vi "Differential Drive Odometry - Delta Angle.vi"(6 "Reset":bool, 9 "Delta Theta":dbl, 10 "Right Distance":dbl, 11 "Left Distance":dbl) -> (3 "Pose":T1)   [LabVIEW 2019]
uses:
  <vilib>/Rock Robotics/WPI/ThirdParty/WPILib Extensions/Geometry/Typedef/Pose2d.ctl
  <vilib>/Rock Robotics/WPI/ThirdParty/WPILib Extensions/Geometry/Typedef/Translation2d.ctl
  <vilib>/Rock Robotics/WPI/ThirdParty/WPILib Extensions/Geometry/Typedef/Rotation2d.ctl
  <vilib>/Analysis/coordinate.llb/2D Cartesian Coordinate Rotation (Scalar).vi
  Odometry Set.vi
  <vilib>/Analysis/NI_AALPro.lvlib
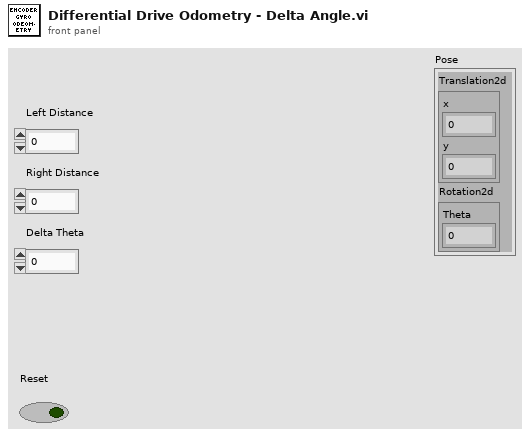
[diagram p1: front panel]
types:
  T1 = typedef "Pose2d.ctl" = cluster{"Translation2d":T2, "Rotation2d":T3}
  T2 = typedef "Translation2d.ctl" = cluster{"x":dbl, "y":dbl}
  T3 = typedef "Rotation2d.ctl" = cluster{"Theta":dbl}
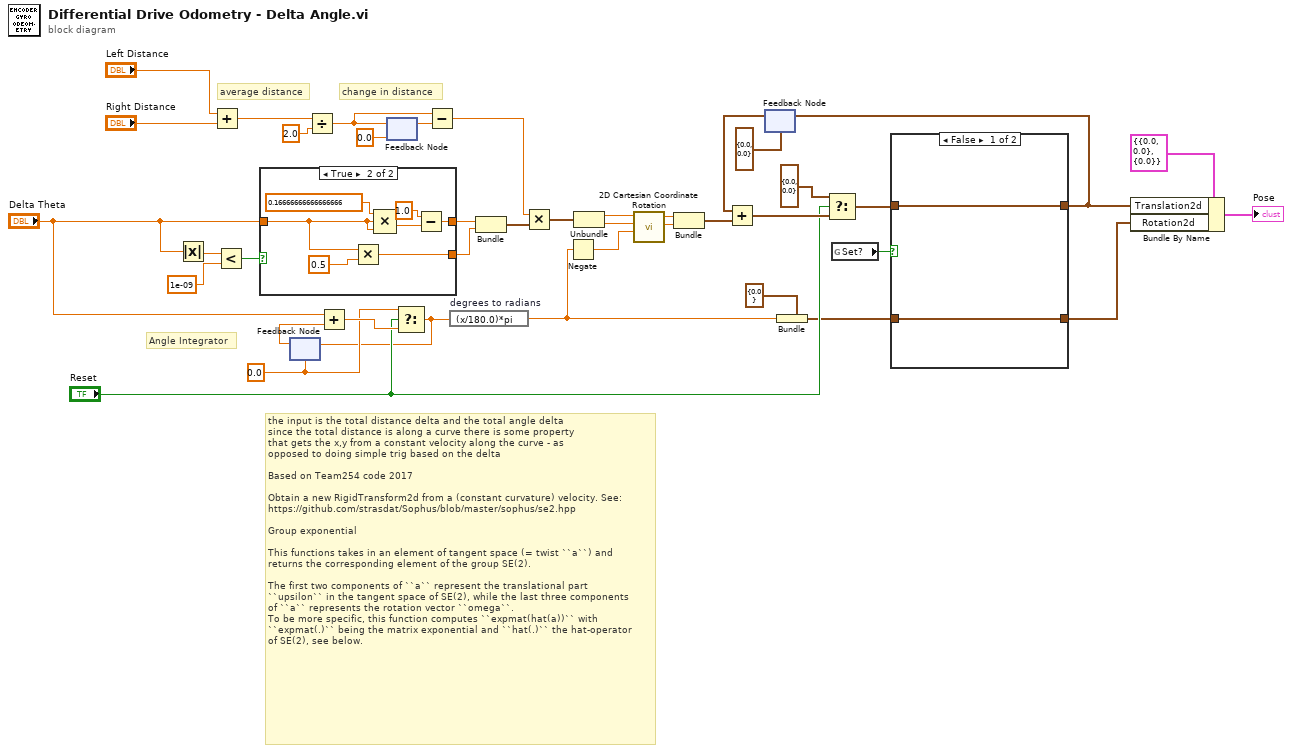
[diagram p0: block diagram]
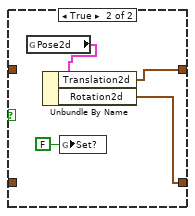
[diagram p2: hidden frame]
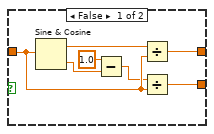
[diagram p3: hidden frame]
diagram:
  w9 = 0.0 ("Delta Theta")
  # "Angle Integrator"
  # "the input is the total distance delta and the total angle delta\nsince the total distance is along a curve there is some property \nthat gets the x,y from a constant velocity along the curve - as\nopposed to doing simple trig based on the delta\n\nBased on Team254 code 2017\n\nObtain a new RigidTransform2d from a (constant curvature) velocity. See:\nhttps://github.com/strasdat/Sophus/blob/master/sophus/se2.hpp\n\nGroup exponential\n\nThis functions takes in an element of tangent space (= twist ``a``) and\nreturns the corresponding element of the group SE(2).\n\nThe first two components of ``a`` represent the translational part\n``upsilon`` in the tangent space of SE(2), while the last three components\nof ``a`` represents the rotation vector ``omega``.\nTo be more specific, this function computes ``expmat(hat(a))`` with\n``expmat(.)`` being the matrix exponential and ``hat(.)`` the hat-operator\nof SE(2), see below."
  # "change in distance"
  # "average distance"
  n1 = Absolute Value(x="Delta Theta") -> (abs(x)=w31:dbl)
  n2 = Add(x="Left Distance", y="Right Distance") -> (x+y=w35:dbl)
  n3 = Less?(x=w31, y=1e-09) -> (x < y?=w29:bool)
  n4 = case shown="True" w29 {
    tunnel: "Delta Theta" -> [w46 w48]
    tunnel: [w42 w49] -> w28
    tunnel: [w41 w53] -> w27
    frame False {
      n5 = Sine & Cosine(0:w46) -> (1:w47:dbl, 2:w44:dbl)
      n6 = Subtract(x=1.0, y=w44) -> (x-y=w43:dbl)
      n7 = Divide(x=w47, y=w46) -> (x/y=w42:dbl)
      n8 = Divide(x=w43, y=w46) -> (x/y=w41:dbl)
    }
    frame True {
      n9 = Multiply(x=w48, y=0.5) -> (x*y=w53:dbl)
      n10 = Compound Arithmetic op=MULTIPLY(0.16666666666666666 ("y"), w48, w48) -> (w52:dbl)
      n11 = Subtract(x=1.0, y=w52) -> (x-y=w49:dbl)
    }
  }
  n12 = feedback #1(w9) -> (w12:dbl)
  n13 = Divide(x=w35, y=2.0) -> (x/y=w34:dbl)
  n14 = Add(x="Delta Theta", y=w12) -> (x+y=w10:dbl)
  n15 = feedback #2(0.0) -> (w40:dbl)
  n16 = feedback-in #2(w34) -> ()
  n17 = Select(t=w9, s="Reset", f=w10) -> (s? t:f=w7:dbl)
  n18 = feedback-in #1(w7) -> ()
  n19 = Subtract(x=w34, y=w40) -> (x-y=w25:dbl)
  n20 = expression code="(x/180.0)*pi" "degrees to radians"(w7) -> (w1:dbl)
  n21 = Bundle(w28, w27) -> (w26:cluster{dbl, dbl})  [unwired: 1 in]
  n22 = Multiply(x=w25, y=w26) -> (x*y=w24:cluster{dbl, dbl})
  n23 = Negate(x=w1) -> (-x=w15:dbl)
  n24 = Unbundle(w24) -> (w23:dbl, w22:dbl)
  n25 = call-poly <vilib>:"2D Cartesian Coordinate Rotation.vi"("theta"=w15, "y"=w22, "x"=w23) -> ("y out"=w20:dbl, "x out"=w21:dbl)  [unwired: 6 in, 1 out]
  n26 = Bundle("x out"=w21, "y out"=w20) -> (w19:cluster{"x out":dbl, "y out":dbl})  [unwired: 1 in]
  n27 = feedback #3(T2 {"x"=0.0, "y"=0.0} ("Translation2d")) -> (w38:T2)
  n28 = Add(x=w38, y=w19) -> (x+y=w32:T2)
  n29 = Bundle(cluster=T3 {"Theta"=0.0} ("Rotation2d"), "Theta"=w1) -> (w3:T3)
  n30 = Select(t=T2 {"x"=0.0, "y"=0.0} ("Translation2d"), s="Reset", f=w32) -> (s? t:f=w5:T2)
  n31 = global read "Odometry Set.vi" "Set?"() -> (w6:bool)
  n32 = case shown="False" w6 {
    tunnel: w5 -> [w56 _]
    tunnel: [w56 w57] -> w4
    tunnel: w3 -> [w55 _]
    tunnel: [w55 w58] -> w2
    frame False {
    }
    frame True {
      n33 = global read "Odometry Set.vi" "Pose2d"() -> (w59:T1)
      n34 = Unbundle By Name(w59) -> ("Translation2d"=w57:T2, "Rotation2d"=w58:T3)
      n35 = global write "Odometry Set.vi" "Set?"(FALSE ("Set?")) -> ()
    }
  }
  n36 = feedback-in #3(w4) -> ()
  n37 = Bundle By Name(cluster=T1 {"Translation2d"={"x"=0.0, "y"=0.0}, "Rotation2d"={"Theta"=0.0}} ("Pose2d"), "Translation2d"=w4, "Rotation2d"=w2) -> (→"Pose":T1)
